vi "Write DAQ DVR FIFO.vi"(6 "FIFO Timestamps":T1, 8 "error in (no error)":errorcluster, 9 "Timeout (ms)":i32=100, 10 "Data In":refnum<data-value>[](array[refnum]), 11 "CIFTag in":refnum<class "CIF_NIChn_Fifo_DAQ.lvclass">) -> (0 "error out":errorcluster, 1 "timed out?":bool, 2 "Data Out":refnum<data-value>[](array[refnum]), 3 "CIFTag out":refnum<class "CIF_NIChn_Fifo_DAQ.lvclass">)   [LabVIEW 2021, in "CIF_NIChn_Fifo_DAQ.lvclass"]
uses:
  CIF_NIChn_Fifo_DAQ.lvclass
  ChannelCommon/typedef/TimeStamps.ctl
  ChannelCommon/ChannelCommon.lvlib
  ChannelCommon/typedef/Datatype Waveform.ctl
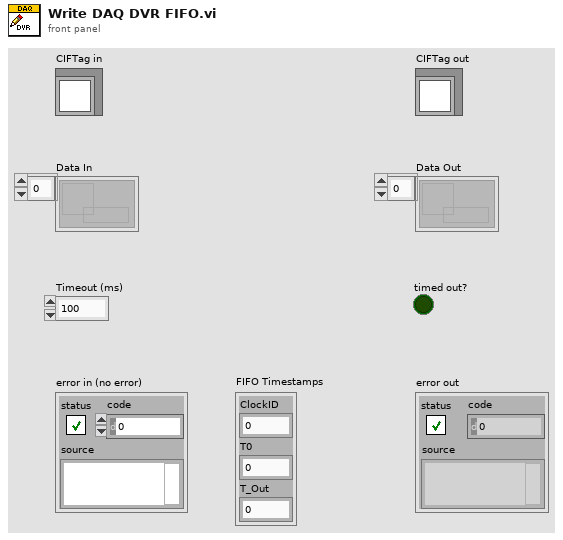
[diagram p1: front panel]
types:
  T1 = typedef "ChannelCommon.lvlib/TimeStamps.ctl" = cluster{"ClockID":u8, "T0":u64, "T_Out":u64}
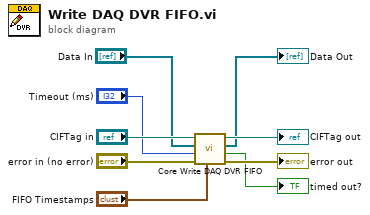
[diagram p0: block diagram]
diagram:
  n1 = call "Core Write DAQ DVR FIFO.vi"("FIFO Timestamps"="FIFO Timestamps", "error in (no error)"="error in (no error)", "Timeout (ms)"="Timeout (ms)", "Data In"="Data In", "CIFTag in"="CIFTag in") -> ("error out"=→"error out":errorcluster, "timed out?"=→"timed out?":bool, "Data Out"=→"Data Out":refnum<data-value>[], "CIFTag out"=→"CIFTag out":refnum<class "CIF_NIChn_Fifo_DAQ.lvclass">)  [unwired: 3 in]
